vi "test Find and Initialize SLSC Switch CD.vi"(8 "error in (no error)":errorcluster, 11 "TestCase in":refnum<class "SLSC Switch Scripting Unit Tests.lvclass">) -> (0 "error out":errorcluster, 3 "TestCase out":refnum<class "SLSC Switch Scripting Unit Tests.lvclass">)   [LabVIEW 2017, in "SLSC Switch Scripting Unit Tests.lvclass"]
uses:
  SLSC Switch Scripting Unit Tests.lvclass
  <vilib>/NI Veristand/Custom Device API/Custom Device Item Ref.ctl
  SLSC Switch Scripting Unit Tests.lvclass/SLSC Switch Scripting Unit Tests.ctl
  Custom Device/Find All SLSC Switch Custom Devices.vi
  Custom Device/Find SLSC Switch Custom Device by Name.vi
  <vilib>/addons/_JKI Toolkits/VI Tester/TestCase.llb/TestCase.lvclass
  SLSC Switch Scripting.lvlib
  <vilib>/NI Veristand/Custom Device API/Custom Device API.lvlib
  Shared/Routing and Faulting Hardware API/Routing and Faulting Hardware API.lvlib
  C:/Program Files (x86)/National Instruments/LabVIEW 2017/vi.lib/addons/_JKI Toolkits/VI Tester/TestCase.llb/TestCase.lvclass
panel:
  in  "Save?":bool
  out "Output Filename":string
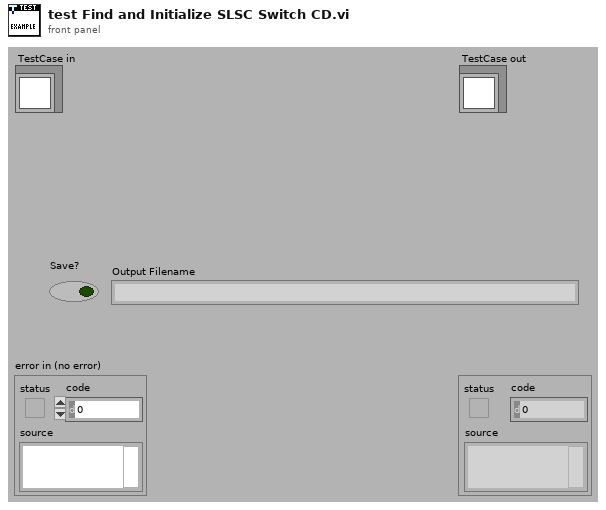
[diagram p1: front panel]
types:
  T1 = typedef "Custom Device API.lvlib/Custom Device Item Ref.ctl" = u64
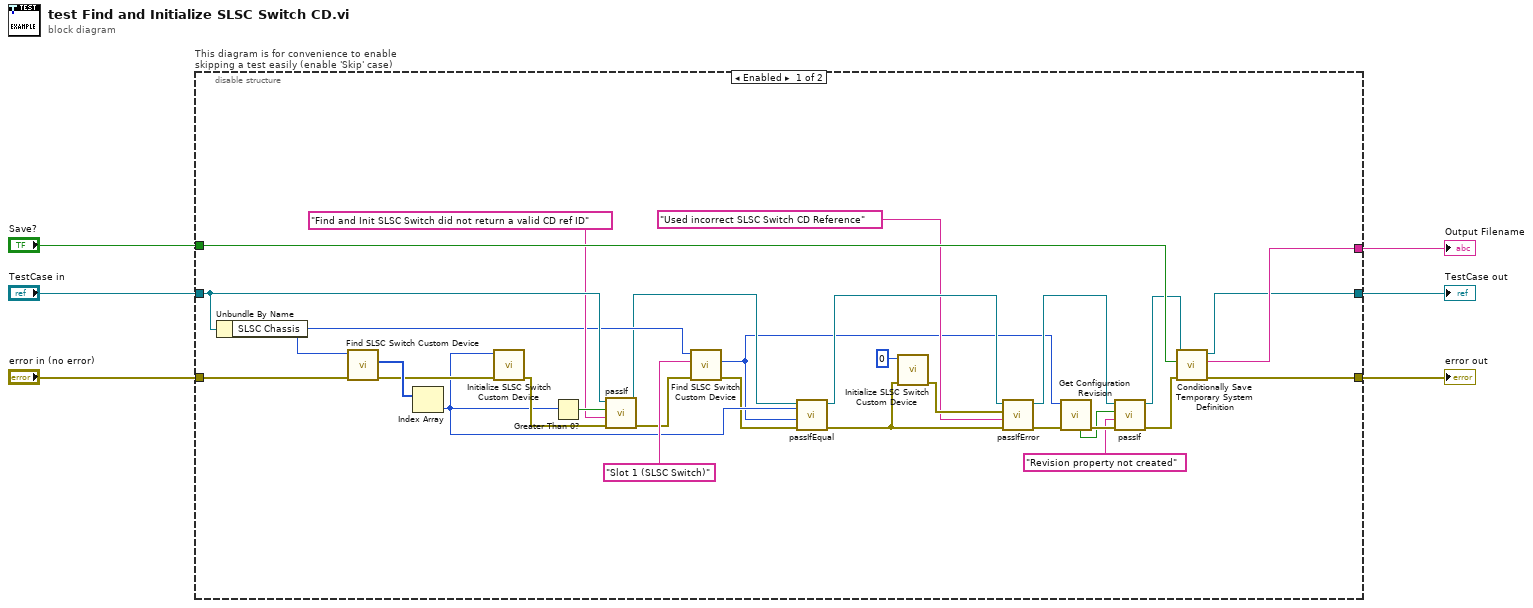
[diagram p0: block diagram]
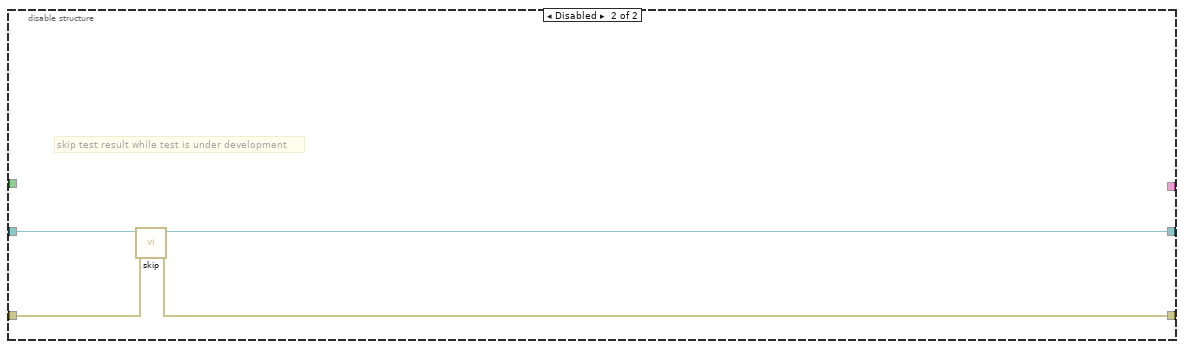
[diagram p2: hidden frame]
diagram:
  n1 = disable-structure "This diagram is for convenience to enable skipping a test easily (enable 'Skip' case)" shown="Enabled" {
    disable-tunnel: "TestCase in" -> [w32 w40]
    disable-tunnel: [w34 w38] -> w3
    disable-tunnel: [w35 w39] -> w5
    disable-tunnel: "error in (no error)" -> [w27 w37]
    disable-tunnel: [w36 _] -> w2
    disable-tunnel: "Save?" -> [w31 _]
    frame Enabled {
      n2 = Unbundle By Name(w32) -> ("SLSC Chassis"=w25:u64)
      n3 = call-poly "Find SLSC Switch Custom Device.vi"("error in (no error)"=w27, "SLSC Chassis Ref"=w25) -> ("error out"=w28:errorcluster, "SLSC Switch Custom Device Ref IDs"=w29:T1[])  [unwired: 7 in, 1 out]
      n4 = Index Array(array=w29) -> (element=w23:T1)  [unwired: 1 in]
      n5 = call "Initialize SLSC Switch Custom Device.vi"("error in (no error)"=w28, "SLSC Switch Custom Device Ref in"=w23) -> ("error out"=w26:errorcluster)  [unwired: 7 in, 2 out]
      n6 = Greater Than 0?(x=w23) -> (x > 0?=w33:bool)
      n7 = call-dynamic "passIf.vi"("error in (no error)"=w26, "message (\"\")"="Find and Init SLSC Switch did not return a valid CD ref ID" ("message (\"\")"), "pass"=w33, "TestCase in"=w32) -> ("error out"=w21:errorcluster, "TestCase out"=w22:refnum<class "SLSC Switch Scripting Unit Tests.lvclass">)  [unwired: 6 in]
      n8 = call-poly "Find SLSC Switch Custom Device.vi"("error in (no error)"=w21, "Name"="Slot 1 (SLSC Switch)", "SLSC Chassis Ref"=w25) -> ("error out"=w20:errorcluster, "SLSC Switch Custom Device Ref"=w9:T1)  [unwired: 6 in, 1 out]
      n9 = call-dynamic "passIfEqual.vi"("error in (no error)"=w20, "y"=w9, "x"=w23, "TestCase in"=w22) -> ("error out"=w16:errorcluster, "TestCase out"=w18:refnum<class "SLSC Switch Scripting Unit Tests.lvclass">)  [unwired: 6 in]
      n10 = call "Initialize SLSC Switch Custom Device.vi"("error in (no error)"=w16, "SLSC Switch Custom Device Ref in"=T1 0) -> ("error out"=w19:errorcluster)  [unwired: 7 in, 2 out]
      n11 = call-dynamic "passIfError.vi"("error in (no error)"=w16, "task (\"\")"="Used incorrect SLSC Switch CD Reference" ("task (\"\")"), "error"=w19, "TestCase in"=w18) -> ("error out"=w11:errorcluster, "TestCase out"=w13:refnum<class "SLSC Switch Scripting Unit Tests.lvclass">)  [unwired: 6 in]
      n12 = call "Get Configuration Revision.vi"("error in (no error)"=w11, "Hardware Ref in"=w9) -> ("error out"=w10:errorcluster, "Found?"=w8:bool)  [unwired: 6 in, 2 out]
      n13 = call-dynamic "passIf.vi"("error in (no error)"=w10, "message (\"\")"="Revision property not created" ("message (\"\")"), "pass"=w8, "TestCase in"=w13) -> ("error out"=w14:errorcluster, "TestCase out"=w12:refnum<class "SLSC Switch Scripting Unit Tests.lvclass">)  [unwired: 6 in]
      n14 = call "Conditionally Save Temporary System Definition.vi"("error in (no error)"=w14, "Save?"=w31, "Test Case"=w12) -> ("error out"=w35:errorcluster, "filename"=w36:string, "Test Case"=w34:refnum<class "SLSC Switch Scripting Unit Tests.lvclass">)  [unwired: 6 in]
    }
    frame Disabled {
      # "skip test result while test is under development"
      n15 = call <vilib>:"skip.vi"("error in (no error)"=w37, "TestCase in"=w40) -> ("error out"=w39:errorcluster, "TestCase out"=w38:refnum<class "SLSC Switch Scripting Unit Tests.lvclass">)  [unwired: 8 in]
    }
  }
  "error out" <- w5
  "TestCase out" <- w3
  "Output Filename" <- w2
